vi "CCD_Exposure 1-D v0.80.vi"(7 "CCD GPIB Address":u16=1, 8 "error in":errorcluster, 9 "Mode":u16(ring) items=["No Over-Exposure Correction", "Over-Exposure Correction", "For Wavelength Calibration"], 10 "Shutter Enabled":bool=TRUE, 11 "Exposuretime (s)":dbl=0.5 format="%.2f") -> (0 "Error Out":errorcluster, 1 "#PixelOverflow":u32, 2 "PixelOverflow":bool, 3 "The Data":dbl[](array[numeric])=[1198.0, 1190.0, 1193.0, 1194.0, 1189.0, 1188.0, 1196.0, 1190.0, 1202.0, 1191.0, 1193.0, 1192.0, 1199.0, 1189.0, 1194.0, 1189.0, 1197.0, 1191.0, 1187.0, 1192.0, 1195.0, 1189.0, 1195.0, 1191.0, 1199.0, 1194.0, 1192.0, 1191.0, 1193.0, 1197.0, 1193.0, 1193.0, 1194.0, 1200.0, 1191.0, 1190.0, 1187.0, 1195.0, 1189.0, 1188.0, 1191.0, 1194.0, 1187.0, 1192.0, 1198.0, 1193.0, 1190.0, 1192.0, 1190.0, 1193.0, 1191.0, 1190.0, 1191.0, 1189.0, 1192.0, 1194.0, 1190.0, 1193.0, 1193.0, 1191.0, 1194.0, 1182.0, 1190.0, 1188.0, 1199.0, 1192.0, 1196.0, 1195.0, 1186.0, 1189.0, 1188.0, 1185.0, 1194.0, 1187.0, 1193.0, 1194.0, 1190.0, 1189.0, 1189.0, 1187.0, 1196.0, 1195.0, 1191.0, 1197.0, 1192.0, 1200.0, 1187.0, 1194.0, 1189.0, 1193.0, 1195.0, 1196.0, 1186.0, 1192.0, 1190.0, 1194.0, 1194.0, 1190.0, 1191.0, 1193.0, 1197.0, 1197.0, 1185.0, 1199.0, 1190.0, 1195.0, 1196.0, 1184.0, 1193.0, 1193.0, 1193.0, 1191.0, 1189.0, 1190.0, 1199.0, 1193.0, 1191.0, 1194.0, 1191.0, 1192.0, 1186.0, 1190.0, 1194.0, 1189.0, 1194.0, 1190.0, 1191.0, 1192.0, 1192.0, 1196.0, 1192.0, 1192.0, 1189.0, 1193.0, 1198.0, 1186.0, 1191.0, 1193.0, 1187.0, 1194.0, 1190.0, 1190.0, 1191.0, 1189.0, 1194.0, 1195.0, 1189.0, 1192.0, 1185.0, 1193.0, 1192.0, 1192.0, 1189.0, 1191.0, 1191.0, 1190.0, 1196.0, 1194.0, 1193.0, 1191.0, 1189.0, 1191.0, 1196.0, 1192.0, 1192.0, 1189.0, 1196.0, 1191.0, 1193.0, 1192.0, 1188.0, 1190.0, 1194.0, 1192.0, 1185.0, 1191.0, 1194.0, 1191.0, 1189.0, 1195.0, 1192.0, 1196.0, 1190.0, 1193.0, 1191.0, 1189.0, 1194.0, 1195.0, 1191.0, 1187.0, 1190.0, 1196.0, 1196.0, 1192.0, 1197.0, 1191.0, 1189.0, 1192.0, 1192.0, 1200.0, 1192.0, 1193.0, 1190.0, 1192.0, 1187.0, 1198.0, 1186.0, 1196.0, 1201.0, 1199.0, 1200.0, 1191.0, 1196.0, 1200.0, 1192.0, 1191.0, 1193.0, 1185.0, 1192.0, 1194.0, 1186.0, 1190.0, 1188.0, 1189.0, 1201.0, 1197.0, 1191.0, 1194.0, 1193.0, 1194.0, 1195.0, 1198.0, 1200.0, 1192.0, 1192.0, 1193.0, 1193.0, 1195.0, 1187.0, 1193.0, 1192.0, 1187.0, 1189.0, 1186.0, 1191.0, 1197.0, 1191.0, 1200.0, 1194.0, 1192.0, 1187.0, 1196.0, 1191.0, 1191.0, 1196.0, 1187.0, 1190.0, 1193.0, 1189.0, 1193.0, 1190.0, 1188.0, 1188.0, 1190.0, 1197.0, 1188.0, 1191.0, 1195.0, 1188.0, 1191.0, 1188.0, 1194.0, 1193.0, 1187.0, 1200.0, 1192.0, 1197.0, 1190.0, 1196.0, 1200.0, 1191.0, 1189.0, 1193.0, 1189.0, 1186.0, 1196.0, 1185.0, 1198.0, 1195.0, 1186.0, 1191.0, 1197.0, 1191.0, 1193.0, 1195.0, 1193.0, 1191.0, 1198.0, 1189.0, 1183.0, 1200.0, 1197.0, 1192.0, 1192.0, 1192.0, 1196.0, 1191.0, 1190.0, 1194.0, 1188.0, 1198.0, 1193.0, 1195.0, 1190.0, 1187.0, 1192.0, 1191.0, 1195.0, 1188.0, 1190.0, 1191.0, 1187.0, 1189.0, 1185.0, 1189.0, 1196.0, 1198.0, 1191.0, 1190.0, 1196.0, 1197.0, 1193.0, 1187.0, 1186.0, 1195.0, 1191.0, 1193.0, 1192.0, 1196.0, 1190.0, 1192.0, 1192.0, 1192.0, 1190.0, 1195.0, 1192.0, 1191.0, 1193.0, 1197.0, 1184.0, 1190.0, 1188.0, 1192.0, 1194.0, 1190.0, 1193.0, 1195.0, 1195.0, 1194.0, 1189.0, 1193.0, 1191.0, 1194.0, 1186.0, 1189.0, 1192.0, 1191.0, 1182.0, 1190.0, 1197.0, 1194.0, 1188.0, 1193.0, 1191.0, 1186.0, 1194.0, 1197.0, 1193.0, 1191.0, 1187.0, 1194.0, 1194.0, 1191.0, 1189.0, 1195.0, 1194.0, 1189.0, 1196.0, 1187.0, 1186.0, 1192.0, 1194.0, 1196.0, 1191.0, 1193.0, 1191.0, 1188.0, 1190.0, 1199.0, 1198.0, 1196.0, 1196.0, 1190.0, 1194.0, 1191.0, 1194.0, 1187.0, 1195.0, 1190.0, 1194.0, 1196.0, 1194.0, 1189.0, 1193.0, 1189.0, 1194.0, 1189.0, 1195.0, 1192.0, 1194.0, 1193.0, 1191.0, 1197.0, 1187.0, 1189.0, 1189.0, 1188.0, 1197.0, 1192.0, 1189.0, 1193.0, 1194.0, 1183.0, 1202.0, 1187.0, 1192.0, 1184.0, 1188.0, 1186.0, 1193.0, 1189.0, 1195.0, 1189.0, 1193.0, 1197.0, 1189.0, 1194.0, 1191.0, 1194.0, 1192.0, 1191.0, 1191.0, 1196.0, 1194.0, 1190.0, 1193.0, 1192.0, 1195.0, 1197.0, 1198.0, 1193.0, 1202.0, 1196.0, 1194.0, 1194.0, 1190.0, 1193.0, 1190.0, 1195.0, 1192.0, 1187.0, 1194.0, 1197.0, 1190.0, 1194.0, 1189.0, 1198.0, 1192.0, 1191.0, 1192.0, 1192.0, 1191.0, 1191.0, 1193.0, 1191.0, 1191.0, 1198.0, 1186.0, 1192.0, 1185.0, 1185.0, 1188.0, 1194.0, 1196.0, 1194.0, 1195.0, 1190.0, 1194.0, 1191.0, 1190.0, 1195.0, 1191.0, 1191.0, 1195.0, 1192.0, 1194.0, 1201.0, 1187.0, 1191.0, 1195.0, 1187.0, 1192.0, 1192.0, 1193.0, 1200.0, 1188.0, 1189.0, 1189.0, 1197.0, 1189.0, 1188.0, 1197.0, 1195.0, 1191.0, 1189.0, 1190.0, 1195.0, 1189.0, 1191.0, 1194.0, 1186.0, 1192.0, 1190.0, 1191.0, 1188.0, 1195.0, 1192.0, 1191.0, 1191.0, 1199.0, 1190.0, 1190.0, 1190.0, 1192.0, 1187.0, 1193.0, 1197.0, 1197.0, 1186.0, 1193.0, 1189.0, 1192.0, 1197.0, 1184.0, 1187.0, 1188.0, 1192.0, 1192.0, 1192.0, 1189.0, 1192.0, 1190.0, 1194.0, 1191.0, 1186.0, 1196.0, 1194.0, 1189.0, 1193.0, 1191.0, 1186.0, 1189.0, 1193.0, 1195.0, 1196.0, 1197.0, 1199.0, 1194.0, 1190.0, 1193.0, 1194.0, 1190.0, 1198.0, 1196.0, 1194.0, 1195.0, 1194.0, 1184.0, 1188.0, 1195.0, 1197.0, 1190.0, 1194.0, 1190.0, 1191.0, 1195.0, 1198.0, 1188.0, 1193.0, 1194.0, 1195.0, 1198.0, 1195.0, 1191.0, 1197.0, 1192.0, 1198.0, 1190.0, 1196.0, 1191.0, 1194.0, 1188.0, 1189.0, 1198.0, 1192.0, 1198.0, 1195.0, 1185.0, 1191.0, 1193.0, 1192.0, 1197.0, 1195.0, 1195.0, 1195.0, 1193.0, 1190.0, 1190.0, 1190.0, 1198.0, 1195.0, 1191.0, 1194.0, 1190.0, 1190.0, 1194.0, 1194.0, 1195.0, 1192.0, 1190.0, 1194.0, 1195.0, 1192.0, 1192.0, 1194.0, 1189.0, 1192.0, 1193.0, 1188.0, 1194.0, 1195.0, 1196.0, 1193.0, 1192.0, 1201.0, 1191.0, 1198.0, 1197.0, 1191.0, 1192.0, 1191.0, 1194.0, 1193.0, 1188.0, 1192.0, 1189.0, 1183.0, 1189.0, 1190.0, 1192.0, 1189.0, 1196.0, 1193.0, 1197.0, 1185.0, 1193.0, 1189.0, 1191.0, 1196.0, 1195.0, 1193.0, 1193.0, 1191.0, 1189.0, 1193.0, 1192.0, 1192.0, 1192.0, 1190.0, 1191.0, 1193.0, 1193.0, 1197.0, 1195.0, 1189.0, 1193.0, 1188.0, 1194.0, 1197.0, 1194.0, 1195.0, 1196.0, 1190.0, 1194.0, 1188.0, 1197.0, 1195.0, 1191.0, 1195.0, 1192.0, 1194.0, 1188.0, 1190.0, 1197.0, 1197.0, 1191.0, 1187.0, 1197.0, 1191.0, 1193.0, 1188.0, 1191.0, 1194.0, 1193.0, 1195.0, 1192.0, 1195.0, 1189.0, 1193.0, 1193.0, 1195.0, 1190.0, 1192.0, 1196.0, 1188.0, 1187.0, 1193.0, 1192.0, 1192.0, 1194.0, 1185.0, 1199.0, 1190.0, 1193.0, 1191.0, 1198.0, 1189.0, 1190.0, 1191.0, 1190.0, 1193.0, 1195.0, 1186.0, 1190.0, 1193.0, 1191.0, 1189.0, 1197.0, 1193.0, 1198.0, 1190.0, 1192.0, 1193.0, 1191.0, 1196.0, 1193.0, 1196.0, 1190.0, 1190.0, 1198.0, 1192.0, 1199.0, 1198.0, 1190.0, 1191.0, 1191.0, 1196.0, 1190.0, 1196.0, 1195.0, 1191.0, 1196.0, 1195.0, 1193.0, 1190.0, 1190.0, 1195.0, 1193.0, 1187.0, 1197.0, 1185.0, 1191.0, 1189.0, 1191.0, 1193.0, 1192.0, 1188.0, 1196.0, 1193.0, 1191.0, 1193.0, 1193.0, 1190.0, 1192.0, 1192.0, 1192.0, 1195.0, 1191.0, 1195.0, 1189.0, 1189.0, 1191.0, 1191.0, 1185.0, 1192.0, 1191.0, 1193.0, 1201.0, 1199.0, 1197.0, 1206.0, 1201.0, 1207.0, 1200.0, 1198.0, 1195.0, 1188.0, 1194.0, 1186.0, 1190.0, 1197.0, 1188.0, 1193.0, 1196.0, 1193.0, 1192.0, 1192.0, 1188.0, 1196.0, 1186.0, 1193.0, 1194.0, 1188.0, 1190.0, 1190.0, 1192.0, 1190.0, 1191.0, 1191.0, 1200.0, 1192.0, 1199.0, 1193.0, 1190.0, 1190.0, 1199.0, 1187.0, 1193.0, 1190.0, 1188.0, 1194.0, 1194.0, 1196.0, 1194.0, 1195.0, 1190.0, 1187.0, 1187.0, 1196.0, 1193.0, 1199.0, 1190.0, 1193.0, 1193.0, 1191.0, 1198.0, 1192.0, 1193.0, 1192.0, 1193.0, 1189.0, 1189.0, 1197.0, 1189.0, 1194.0, 1193.0, 1192.0, 1185.0, 1198.0, 1193.0, 1189.0, 1192.0, 1193.0, 1196.0, 1190.0, 1195.0, 1189.0, 1196.0, 1198.0, 1190.0, 1191.0, 1193.0, 1186.0, 1189.0, 1195.0, 1188.0, 1197.0, 1188.0, 1191.0, 1185.0, 1190.0, 1193.0, 1188.0, 1198.0, 1192.0, 1193.0, 1194.0, 1194.0, 1189.0, 1184.0, 1193.0, 1199.0, 1193.0, 1192.0, 1193.0, 1190.0, 1196.0, 1191.0, 1192.0, 1189.0, 1194.0, 1188.0, 1189.0, 1190.0, 1190.0, 1192.0, 1195.0, 1188.0, 1190.0, 1192.0, 1189.0, 1197.0, 1192.0, 1194.0, 1187.0, 1196.0, 1192.0, 1194.0, 1185.0, 1187.0, 1187.0, 1191.0, 1195.0, 1190.0, 1186.0, 1183.0, 1194.0, 1194.0, 1192.0, 1192.0, 1188.0, 1193.0, 1195.0, 1189.0, 1190.0, 1191.0, 1192.0, 1196.0, 1186.0, 1195.0, 1191.0, 1185.0, 1191.0, 1187.0, 1190.0, 1188.0, 1189.0, 1187.0, 1196.0, 1191.0, 1190.0, 1191.0, 1190.0, 1196.0, 1195.0, 1186.0, 1187.0, 1187.0, 1188.0, 1194.0, 1192.0, 1192.0, 1192.0, 1189.0, 1192.0, 1191.0, 1188.0, 1188.0, 1187.0, 1187.0, 1190.0, 1186.0, 1191.0, 1195.0, 1192.0, 1196.0, 1193.0, 1192.0, 1191.0, 1189.0, 1187.0, 1193.0, 1188.0, 1189.0, 1194.0, 1191.0, 1185.0, 1193.0, 1191.0, 1196.0, 1196.0, 1199.0, 1195.0, 1211.0] format="%.2f", 4 "GPIB Status":i16=-1, 5 "Exposuretime (s) out":dbl format="%.2f", 6 "Setup String":string="ldu,0,256,16;sdu,0,1024,1024;cl0;omrm;sron")   [LabVIEW 2021]
uses:
  Globals and TypeDefs/Global Varibal Control.vi
panel:
  out "Array Length":i32=1024
  out "Plot":i32[](graph)
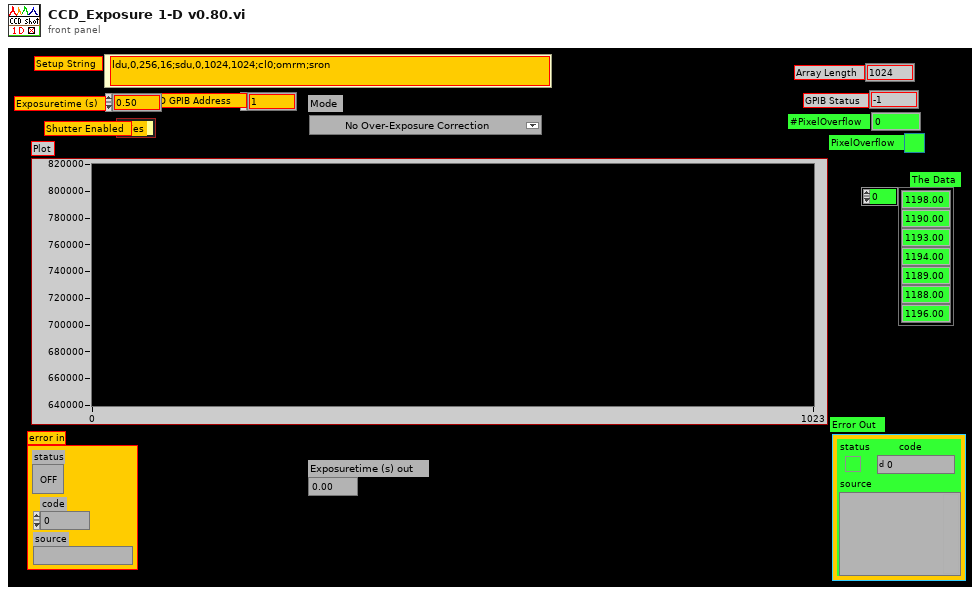
[diagram p1: front panel]
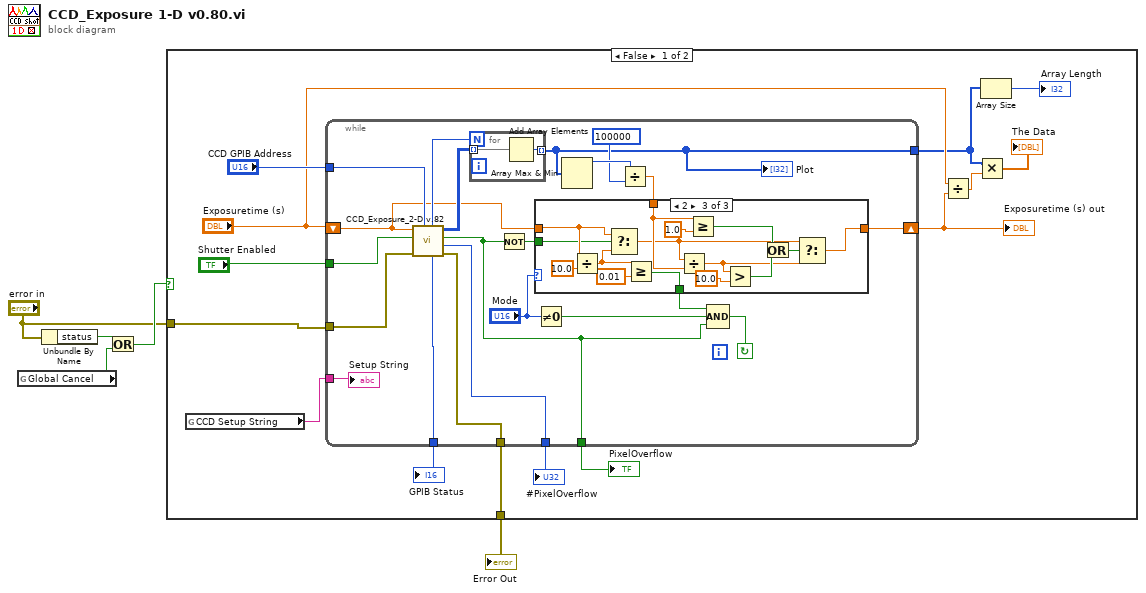
[diagram p0: block diagram]
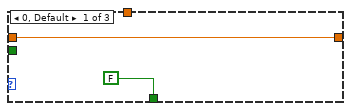
[diagram p2: hidden frame]
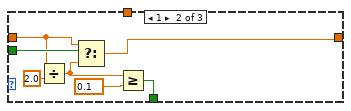
[diagram p3: hidden frame]
diagram:
  n1 = global read "Global Varibal Control.vi" "Global Cancel"() -> (w1:bool)
  n2 = Unbundle By Name("error in") -> ("status"=w5:bool)
  n3 = Or(x=w5, y=w1) -> (x .or. y?=w4:bool)
  n4 = case shown="False" w4 {
    tunnel: "error in" -> [w8 w67]
    tunnel: [w7 w67] -> w2
    frame False {
      n5 = global read "Global Varibal Control.vi" "CCD Setup String"() -> (w6:string)
      n6 = while {
        tunnel: w6 -> [w20]
        tunnel: [w21] -> w9
        tunnel: [w22] -> w15
        tunnel: [w23] -> w16
        tunnel: [w24] -> w7
        tunnel: [w25] -> w17
        tunnel: "CCD GPIB Address" -> [w35]
        shift-left: "Exposuretime (s)" -> [w33]
        shift-right: [w26] -> w13
        tunnel: w8 -> [w37]
        tunnel: "Shutter Enabled" -> [w38]
        stop <- w36 continue-if-true
        n7 = call "CCD_Exposure_2-D v.82.vi"("CCD GPIB Address"=w35, "error in"=w37, "Shutter Enabled"=w38, "Exposuretime (s)"=w33) -> ("Error Out"=w24:errorcluster, "#PixelOverflow"=w23:u32, "PixelOverflow"=w22:bool, "The Data"=w40:i32[][], "GPIB Status"=w25:i16, "sd"=w39:i32)  [unwired: 1 in, 1 out]
        n8 = for {
          N: w39 -> [_]
          tunnel: [w66] -> w21 mode=indexing
          tunnel: w40 -> [w65] mode=indexing
          n9 = Add Array Elements(numeric array=w65) -> (sum=w66:i32)
        }
        "Plot" <- w21
        n10 = Not(x=w22) -> (.not. x?=w30:bool)
        n11 = Not Equal To 0?(x="Mode") -> (x != 0?=w32:bool)
        n12 = Array Max & Min(array=w21) -> (max value=w29:i32)  [unwired: 3 out]
        n13 = Divide(x=w29, y=100000) -> (x/y=w27:dbl)
        n14 = case shown="2" "Mode" {
          tunnel: [w42 w43 w50] -> w26
          tunnel: w33 -> [w42 w45 w61]
          tunnel: [FALSE w47 w59] -> w31
          tunnel: w30 -> [_ w46 w60]
          tunnel: w27 -> [_ _ w57]
          frame 0, Default {
          }
          frame 1 {
            n15 = Divide(x=w45, y=2.0) -> (x/y=w44:dbl)
            n16 = Select(t=w45, s=w46, f=w44) -> (s? t:f=w43:dbl)
            n17 = Greater Or Equal?(x=w44, y=0.1) -> (x >= y?=w47:bool)
          }
          frame 2 {
            n18 = Divide(x=w61, y=10.0) -> (x/y=w62:dbl)
            n19 = Select(t=w61, s=w60, f=w62) -> (s? t:f=w52:dbl)
            n20 = Greater Or Equal?(x=w62, y=0.01) -> (x >= y?=w59:bool)
            n21 = Divide(x=w52, y=w57) -> (x/y=w51:dbl)
            n22 = Greater Or Equal?(x=w57, y=1.0) -> (x >= y?=w54:bool)
            n23 = Greater?(x=w51, y=10.0) -> (0:w55:bool)
            n24 = Or(x=w54, y=w55) -> (x .or. y?=w53:bool)
            n25 = Select(t=w52, s=w53, f=w51) -> (s? t:f=w50:dbl)
          }
        }
        n26 = Compound Arithmetic op=AND(w31, w32, w22) -> (w36:bool)
        "Setup String" <- w20
      }
      "PixelOverflow" <- w15
      "#PixelOverflow" <- w16
      "GPIB Status" <- w17
      "Exposuretime (s) out" <- w13
      n27 = Divide(x="Exposuretime (s)", y=w13) -> (x/y=w12:dbl)
      n28 = Multiply(x=w9, y=w12) -> (x*y=→"The Data":dbl[])
      n29 = Array Size(array=w9) -> (size(s)=→"Array Length":i32)
    }
    frame True {
    }
  }
  "Error Out" <- w2
